vi "standalone resonant correction.vi"(0 "uncorrected images in":i16[][][](array[numeric]), 1 "resonant.correction.enable":bool, 2 "force reset shift registers":bool, 7 "frames.p.queue.item":dbl, 9 "x.pixels":dbl, 11 "y.pixels":dbl, 12 "x.correction":dbl, 13 "no.of.channels":dbl) -> (4 "corrected images out":i16[][][](array[numeric]))   [LabVIEW 2012]
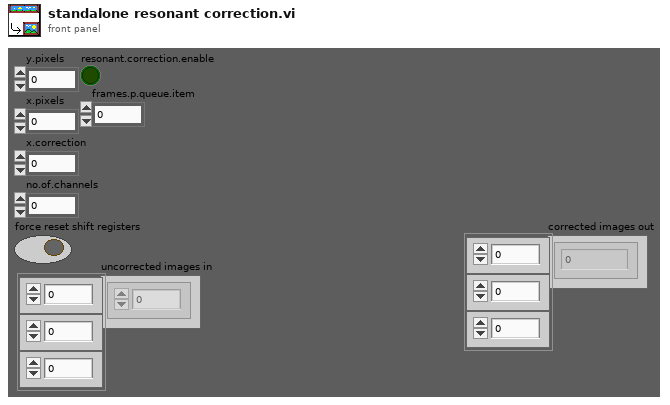
[diagram p1: front panel]
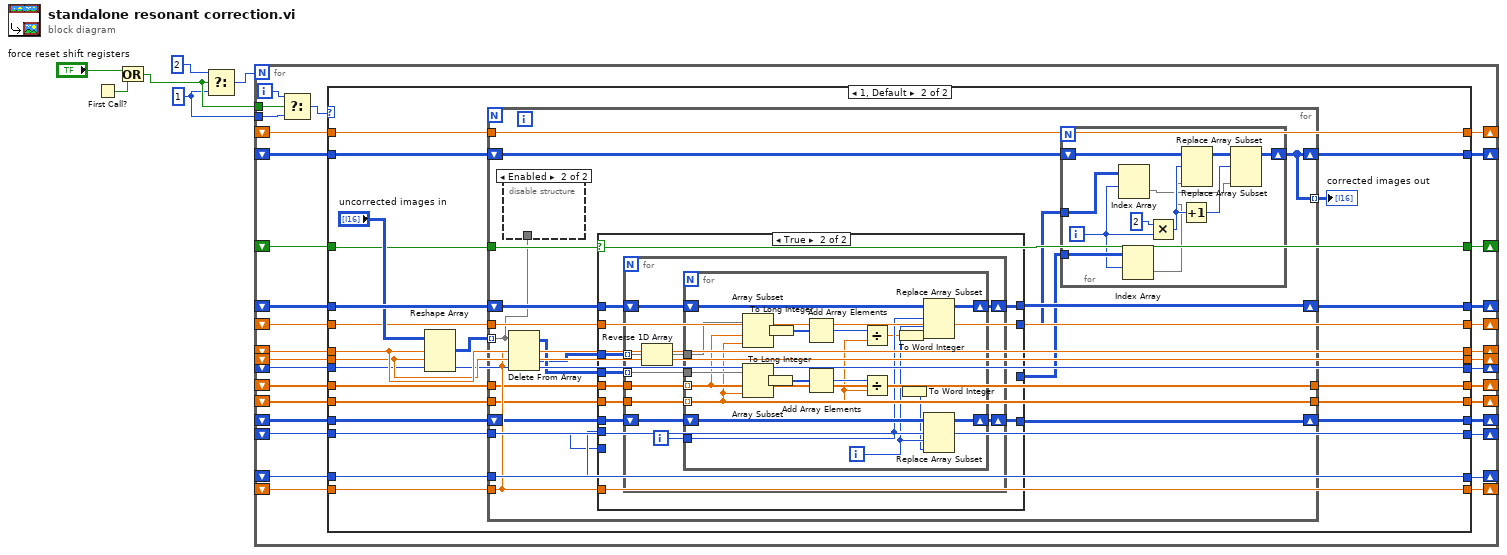
[diagram p0: block diagram]
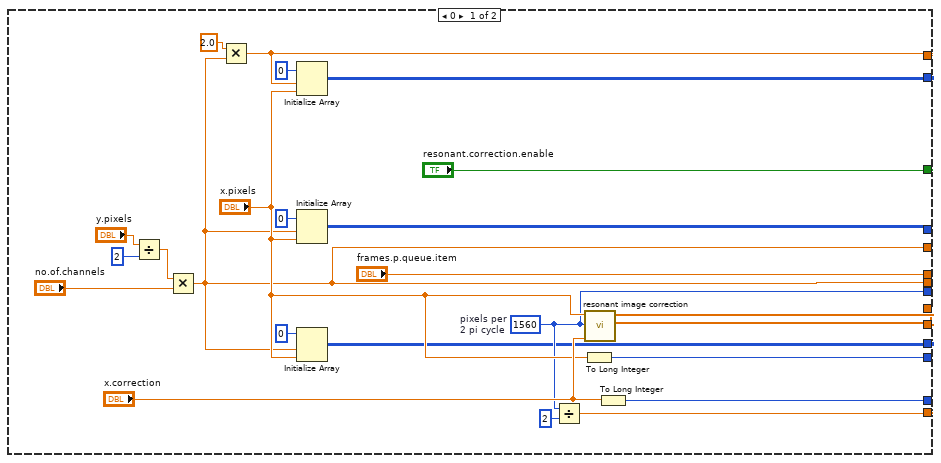
[diagram p2: hidden frame]
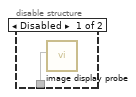
[diagram p3: hidden frame]
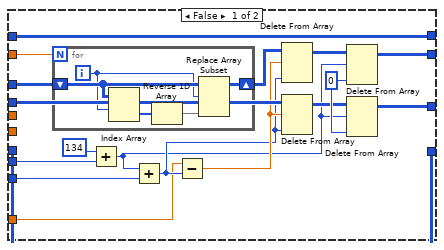
[diagram p4: hidden frame]
diagram:
  w1 = i16 1 ("sum")
  n1 = First Call?() -> (First Call?: T/F=w5:bool)
  n2 = Or(x="force reset shift registers", y=w5) -> (x .or. y?=w2:bool)
  n3 = Select(t=i16 2 ("sum"), s=w2, f=w1) -> (s? t:f=w3:i16)
  n4 = for {
    N: w3 -> [_]
    shift-right: [w29] -> _
    shift-left: _ -> [w35]
    shift-right: [w30] -> _
    shift-left: _ -> [w34]
    shift-right: [w23] -> _
    shift-left: _ -> [w24]
    shift-right: [w21] -> _
    shift-left: _ -> [w33]
    shift-right: [w20] -> _
    shift-left: _ -> [w32]
    shift-right: [w18] -> _
    shift-left: _ -> [w22]
    shift-right: [w16] -> _
    shift-left: _ -> [w36]
    shift-right: [w15] -> _
    shift-left: _ -> [w25]
    shift-right: [w14] -> _
    shift-left: _ -> [w27]
    shift-right: [w12] -> _
    shift-left: _ -> [w38]
    shift-right: [w13] -> _
    shift-left: _ -> [w26]
    shift-right: [w17] -> _
    shift-left: _ -> [w28]
    shift-right: [w11] -> _
    shift-left: _ -> [w31]
    shift-right: [w19] -> _
    shift-left: _ -> [w37]
    tunnel: w2 -> [w9]
    tunnel: w1 -> [w8]
    i -> [w10]
    n5 = Select(t=w10, s=w9, f=w8) -> (s? t:f=w7:i32)
    n6 = case shown="1, Default" w7 {
      tunnel: w38 -> [_ w63]
      tunnel: w37 -> [_ w71]
      tunnel: w36 -> [_ w68]
      tunnel: w35 -> [_ w84]
      tunnel: w34 -> [_ w83]
      tunnel: w33 -> [_ w82]
      tunnel: w32 -> [_ w81]
      tunnel: w31 -> [_ w67]
      tunnel: [w43 w80] -> w30
      tunnel: [w49 w79] -> w29
      tunnel: w28 -> [_ w69]
      tunnel: w27 -> [_ w65]
      tunnel: w26 -> [_ w64]
      tunnel: w25 -> [_ w66]
      tunnel: w24 -> [_ w78]
      tunnel: [w51 w77] -> w23
      tunnel: w22 -> [_ w70]
      tunnel: [w44 w73] -> w21
      tunnel: [w45 w72] -> w20
      tunnel: [w41 w71] -> w19
      tunnel: [w52 w70] -> w18
      tunnel: [w42 w69] -> w17
      tunnel: ["resonant.correction.enable" w68] -> w16
      tunnel: [w39 w66] -> w15
      tunnel: ["frames.p.queue.item" w65] -> w14
      tunnel: [w39 w64] -> w13
      tunnel: [w46 w63] -> w12
      tunnel: [w40 w67] -> w11
      frame 0 {
        w46 = 1560  # pixels per 2 pi cycle
        n7 = Divide(x="y.pixels", y=2) -> (x/y=w48:dbl)
        n8 = Multiply(x=w48, y="no.of.channels") -> (x*y=w39:dbl)
        n9 = Multiply(x=2.0, y=w39) -> (x*y=w52:dbl)
        n10 = Initialize Array(i16 0 ("sum"), w52, "x.pixels") -> (w51:i16[][])
        n11 = Initialize Array(i16 0 ("sum"), w39, "x.pixels") -> (w49:i16[][])
        n12 = Initialize Array(i16 0 ("sum"), w39, "x.pixels") -> (w43:i16[][])
        n13 = Divide(x=w46, y=2) -> (x/y=w41:dbl)
        n14 = To Long Integer(number="x.pixels") -> (32bit integer=w42:i32)
        n15 = call "resonant image correction.vi"("shift index"="x.correction", "pixels per period (2pi, 2 lines)"=w46, "x pixels"="x.pixels") -> ("histogram cumsum"=w44:dbl[], "histogram pixels to avg"=w45:dbl[])  [unwired: 7 in]
        n16 = To Long Integer(number="x.correction") -> (32bit integer=w40:i32)
      }
      frame 1, Default {
        n17 = Reshape Array("uncorrected images in", w65, w64, w63) -> (w76:i16[][][])
        n18 = for {
          tunnel: w76 -> [w85] mode=indexing
          tunnel: w71 -> [w103]
          tunnel: w68 -> [w102]
          tunnel: w82 -> [w87]
          tunnel: w81 -> [w86]
          tunnel: w67 -> [w99]
          shift-right: [w98] -> w80
          shift-left: w83 -> [w100]
          shift-right: [w97] -> w79
          shift-left: w84 -> [w101]
          tunnel: w69 -> [w96]
          tunnel: w66 -> [w95]
          shift-right: [w93] -> w77
          shift-left: w78 -> [w94]
          tunnel: w70 -> [w92]
          tunnel: [w93] -> w75 mode=indexing
          tunnel: [w87] -> w73
          tunnel: [w86] -> w72
          n19 = disable-structure shown="Enabled" {
            disable-tunnel: w85 -> [w104 _]
            frame Disabled {
              n20 = call "image display probe.vi"("Image Pixels (I16)"=w104) -> ()  [unwired: 11 in]
            }
            frame Enabled {
            }
          }
          n21 = Delete From Array(array=w85, length=w103, index (col)=w103) -> (deleted portion=w90:i16[][], array with subset deleted=w91:i16[][])  [unwired: 1 in]
          n22 = case shown="True" w102 {
            tunnel: w90 -> [w108 w135]
            tunnel: w91 -> [w119 w134]
            tunnel: w87 -> [_ w133]
            tunnel: w86 -> [_ w132]
            tunnel: w101 -> [w120 w131]
            tunnel: w100 -> [w106 w130]
            tunnel: [w117 w129] -> w88
            tunnel: [w115 w128] -> w89
            tunnel: w99 -> [w121 _]
            tunnel: [w106 w129] -> w98
            tunnel: [w120 w128] -> w97
            tunnel: w96 -> [w114 _]
            tunnel: w95 -> [w109 _]
            tunnel: w103 -> [w107 _]
            frame False {
              w122 = 0 ("disabled index (col)")
              n23 = for {
                N: w109 -> [_]
                shift-right: [w126] -> w105
                shift-left: w108 -> [w125]
                i -> [w124]
                n24 = Index Array(array=w125, index (row)=w124) -> (element=w123:i16[])  [unwired: 1 in]
                n25 = Reverse 1D Array(array=w123) -> (reversed array=w127:i16[])
                n26 = Replace Array Subset(array=w125, new element=w127, index (row)=w124) -> (w126:i16[][])  [unwired: 1 in]
              }
              n27 = Add(x=134 ("length"), y=w121) -> (x+y=w110:i32)
              n28 = Add(x=w110, y=w114) -> (x+y=w111:i32)
              n29 = Subtract(x=w107, y=w111) -> (x-y=w112:dbl)
              n30 = Delete From Array(array=w105, length=w112, index (col)=w111) -> (array with subset deleted=w116:i16[][])  [unwired: 1 in, 1 out]
              n31 = Delete From Array(array=w119, length=w112, index (col)=w111) -> (array with subset deleted=w118:i16[][])  [unwired: 1 in, 1 out]
              n32 = Delete From Array(array=w116, length=w110, index (col)=w122) -> (array with subset deleted=w115:i16[][])  [unwired: 1 in, 1 out]
              n33 = Delete From Array(array=w118, length=w110, index (col)=w122) -> (array with subset deleted=w117:i16[][])  [unwired: 1 in, 1 out]
            }
            frame True {
              n34 = for {
                tunnel: w135 -> [w143] mode=indexing
                tunnel: w134 -> [w142] mode=indexing
                tunnel: w133 -> [w145]
                tunnel: w132 -> [w144]
                shift-right: [w137] -> w128
                shift-left: w131 -> [w141]
                shift-right: [w138] -> w129
                shift-left: w130 -> [w140]
                i -> [w139]
                n35 = Reverse 1D Array(array=w143) -> (reversed array=w136:i16[])
                n36 = for {
                  tunnel: w145 -> [w164] mode=indexing
                  tunnel: w144 -> [w159] mode=indexing
                  tunnel: w136 -> [w150]
                  tunnel: w142 -> [w165]
                  shift-right: [w152] -> w137
                  shift-left: w141 -> [w156]
                  shift-right: [w153] -> w138
                  shift-left: w140 -> [w157]
                  tunnel: w139 -> [w155]
                  i -> [w151]
                  n37 = Array Subset(array=w150, index=w164, length=w159) -> (w162:i16[])
                  n38 = Array Subset(array=w165, index=w164, length=w159) -> (w163:i16[])
                  n39 = To Long Integer(number=w163) -> (32bit integer=w148:i32[])
                  n40 = To Long Integer(number=w162) -> (32bit integer=w149:i32[])
                  n41 = Add Array Elements(numeric array=w149) -> (sum=w160:i32)
                  n42 = Add Array Elements(numeric array=w148) -> (sum=w161:i32)
                  n43 = Divide(x=w160, y=w159) -> (x/y=w154:dbl)
                  n44 = Divide(x=w161, y=w159) -> (x/y=w158:dbl)
                  n45 = To Word Integer(number=w154) -> (16bit integer=w147:i16)
                  n46 = To Word Integer(number=w158) -> (16bit integer=w146:i16)
                  n47 = Replace Array Subset(array=w156, new element=w147, index (row)=w155, index (col)=w151) -> (w152:i16[][])
                  n48 = Replace Array Subset(array=w157, new element=w146, index (row)=w155, index (col)=w151) -> (w153:i16[][])
                }
              }
            }
          }
          n49 = for {
            N: w92 -> [_]
            shift-right: [w172] -> w93
            shift-left: w94 -> [w174]
            tunnel: w89 -> [w176]
            tunnel: w88 -> [w175]
            i -> [w169]
            n50 = Index Array(array=w176, index (row)=w169) -> (element=w166:i16[])  [unwired: 1 in]
            n51 = Index Array(array=w175, index (row)=w169) -> (element=w167:i16[])  [unwired: 1 in]
            n52 = Multiply(x=2, y=w169) -> (x*y=w168:i32)
            n53 = Increment(x=w168) -> (x+1=w170:i32)
            n54 = Replace Array Subset(array=w174, new element=w167, index (row)=w168) -> (w173:i16[][])  [unwired: 1 in]
            n55 = Replace Array Subset(array=w173, new element=w166, index (row)=w170) -> (w172:i16[][])  [unwired: 1 in]
          }
        }
        "corrected images out" <- w75
      }
    }
  }
